vi "Force Quit LabVIEW.vi"(8 "error in":errorcluster, 9 "Exit Code (0)":u32, 10 "Quit (T)":bool=TRUE) -> (0 "error out":errorcluster, 3 "Quit Successfully":bool)   [LabVIEW 2016, in "数据传输系统-06.lvlib"]
doc: "Force-quit current application via WinAPI. \n\nWARNING: This VI will exit LabView immediately when run, without saving anything!"
uses:
  kernel32.dll
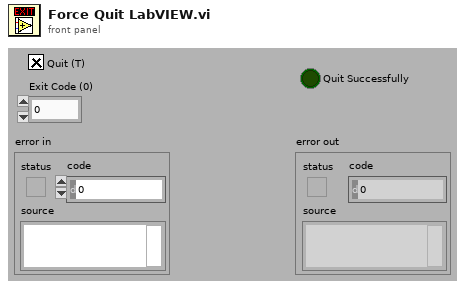
[diagram p1: front panel]
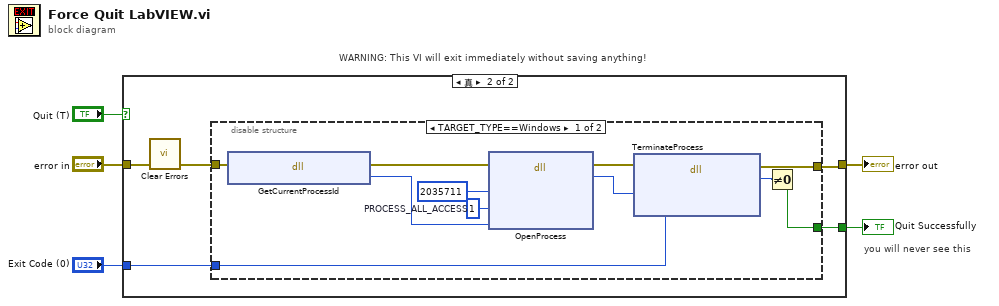
[diagram p0: block diagram]
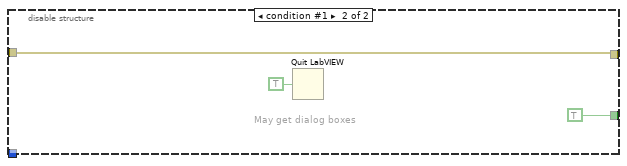
[diagram p3: hidden frame]
diagram:
  # "WARNING: This VI will exit immediately without saving anything!"
  # "you will never see this"
  n1 = case shown="真" "Quit (T)" {
    tunnel: [w6 w11] -> w5
    tunnel: [_ w10] -> w4
    tunnel: "error in" -> [w6 w9]
    tunnel: "Exit Code (0)" -> [_ w7]
    frame False {
    }
    frame True {
      n2 = call <vilib>:"Clear Errors.vi"("error in (no error)"=w9) -> ("error out"=w8:errorcluster)  [unwired: 5 in, 1 out]
      n3 = disable-structure shown="TARGET_TYPE==Windows" {
        disable-tunnel: [w18 w23] -> w11
        disable-tunnel: [w17 TRUE ("quit? (T)")] -> w10
        disable-tunnel: w8 -> [w13 w23]
        disable-tunnel: w7 -> [w12 _]
        frame condition #0 (active) {
          w21 = 2035711  # PROCESS_ALL_ACCESS
          n4 = dll-call lib="kernel32.dll" fn="GetCurrentProcessId"(error in=w13) -> (error out=w15:errorcluster, "dwProcessID"=w14:i32)  [unwired: 2 in, 1 out]
          n5 = dll-call lib="kernel32.dll" fn="OpenProcess"(error in=w15, "dwDesiredAccess"=w21, "bInheritHandle"=1, "dwProcessID"=w14) -> (error out=w20:errorcluster, "hProcess"=w16:i32)  [unwired: 2 in, 4 out]
          n6 = dll-call lib="kernel32.dll" fn="TerminateProcess"(error in=w20, "hProcess"=w16, "uExitCode"=w12) -> (error out=w18:errorcluster, "BoolSuccess"=w19:i32)  [unwired: 2 in, 3 out]
          n7 = Not Equal To 0?(x=w19) -> (x != 0?=w17:bool)
        }
        frame condition #1 {
          # "May get dialog boxes"
          n8 = Quit LabVIEW(quit? (T)=TRUE) -> ()
        }
      }
    }
  }
  "error out" <- w5
  "Quit Successfully" <- w4
